vi "Utility Multiple Write To Registers.vi"(6 "Direct Action?":bool, 7 "Unit Address (1)":u8=1, 8 "error in (no error)":errorcluster, 9 "Array Of Data":i16[](array[numeric]), 10 "Register Address (0)":u16, 11 "VISA resource name":refnum<visa-resource-name>) -> (0 "error out":errorcluster, 3 "VISA resource name out":refnum<visa-resource-name>)   [LabVIEW 2010]
doc: "This VI writes the values to the specified registers of specified unit."
uses:
  MBDRV_Command Data.ctl
  MBDRV_Action.ctl
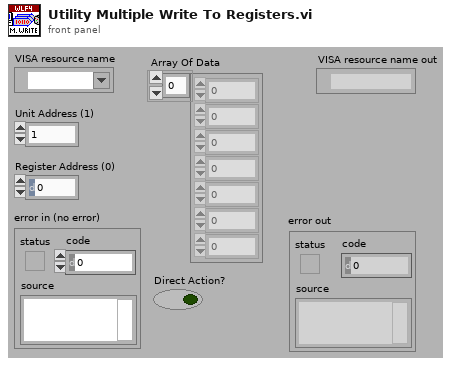
[diagram p1: front panel]
types:
  T1 = typedef "MBDRV_Action.ctl" = enum16{"Write", "Read"}
  T2 = typedef "MBDRV_Command Data.ctl" = cluster{"Action":T1, "Com Port":string, "Register Address":u16, "Data To Write/Num To Read":i16}
  T3 = enum16{"By The Number of Bytes", "Copy Of the Sent Message"}
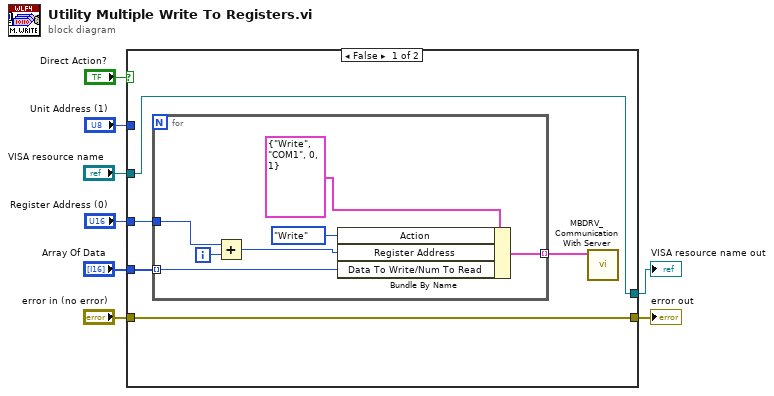
[diagram p0: block diagram]
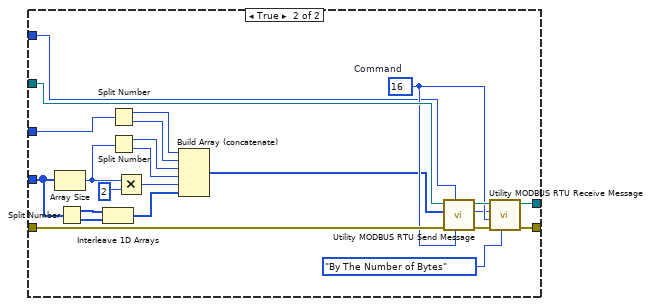
[diagram p2: hidden frame]
diagram:
  n1 = case shown="False" "Direct Action?" {
    tunnel: "VISA resource name" -> [w13 w43]
    tunnel: [w13 w42] -> w7
    tunnel: "error in (no error)" -> [w12 w41]
    tunnel: [w12 w30] -> w5
    tunnel: "Unit Address (1)" -> [_ w29]
    tunnel: "Register Address (0)" -> [w10 w26]
    tunnel: "Array Of Data" -> [w11 w25]
    frame False {
      n2 = for {
        tunnel: w11 -> [w14] mode=indexing
        tunnel: w10 -> [w16]
        tunnel: [w19] -> w9 mode=indexing
        i -> [w17]
        n3 = Add(x=w16, y=w17) -> (x+y=w15:i32)
        n4 = Bundle By Name(cluster=T2 {"Action"=enum."Write", "Com Port"="COM1", "Register Address"=0, "Data To Write/Num To Read"=1} ("Command"), "Action"=MBDRV_Action."Write", "Register Address"=w15, "Data To Write/Num To Read"=w14) -> (w19:T2)
      }
      n5 = call "MBDRV_Communication With Server.vi"("Write To PLC"=w9) -> ()  [unwired: 9 in, 2 out]
    }
    frame True {
      w38 = u8 16  # Command
      n6 = Array Size(array=w25) -> (size(s)=w28:i32)
      n7 = Split Number(x=w25) -> (hi(x)=w22:u8[], lo(x)=w23:u8[])
      n8 = Interleave 1D Arrays(w22, w23) -> (w21:u8[])
      n9 = Split Number(x=w26) -> (hi(x)=w36:u8, lo(x)=w35:u8)
      n10 = Split Number(x=w28) -> (hi(x)=w34:u16, lo(x)=w33:u16)
      n11 = Multiply(x=w28, y=2) -> (x*y=w27:i32)
      n12 = Build Array (concatenate)(w36, w35, w34, w33, w27, w21) -> (w37:i32[])
      n13 = call "Utility MODBUS RTU Send Message.vi"("Command (0)"=w38, "Unit Address (1)"=w29, "error in (no error)"=w41, "Message (empty array)"=w37, "VISA resource name"=w43) -> ("error out"=w40:errorcluster, "Length Of Sent MSG"=w32:u8, "VISA resource name out"=w39:refnum<visa-resource-name>)  [unwired: 4 in]
      n14 = call "Utility MODBUS RTU Receive Message.vi"("Receive Message Type (0: By The Number Of Bytes)"=T3."By The Number of Bytes" ("Receive Message Type"), "error in (no error)"=w40, "Sent Command (0)"=w38, "Length Of Sent MSG (0)"=w32, "VISA resource name"=w39) -> ("error out"=w30:errorcluster, "VISA resource name out"=w42:refnum<visa-resource-name>)  [unwired: 4 in, 1 out]
    }
  }
  "error out" <- w5
  "VISA resource name out" <- w7
